vi "Read turn.vi"(11 "Position in":refnum<class "Position.lvclass">) -> (2 "Turn":T1, 3 "Position out":refnum<class "Position.lvclass">)   [LabVIEW 2016, in "Chesslib.lvlib" / "Position.lvclass"]
uses:
  Position.lvclass
  typedef/Color.ctl
  Position.lvclass/Position.ctl
  Chesslib.lvlib
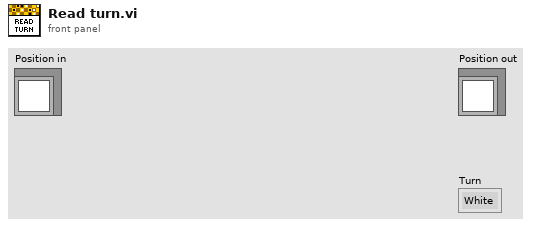
[diagram p1: front panel]
types:
  T1 = typedef "Chesslib.lvlib/Color.ctl" = enum16{"White", "Black"}
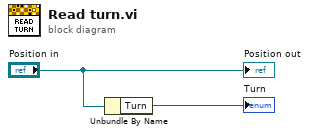
[diagram p0: block diagram]
diagram:
  n1 = Unbundle By Name("Position in") -> ("Turn"=→"Turn":T1)
  "Position out" <- "Position in"
